vi "DAQNavi Read (Counter 1D Count Value NChan 1Samp).vi"(8 "error in (no error)":errorcluster, 11 "task in":i32) -> (0 "error out":errorcluster, 2 "data":i32[](array[numeric]), 3 "task out":i32)   [LabVIEW 2020]
uses:
  DAQNavi_LV.dll
panel:
  in  "timeout":dbl=10.0
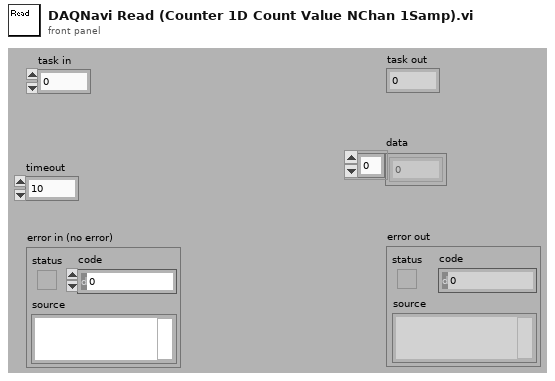
[diagram p1: front panel]
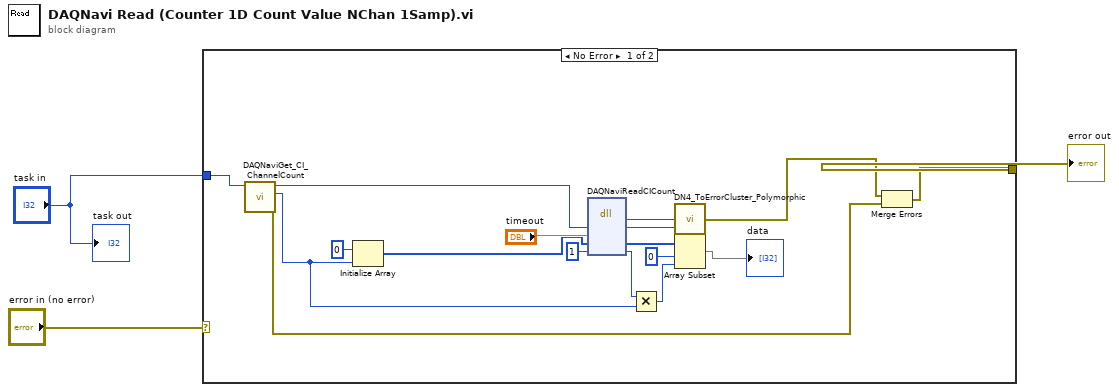
[diagram p0: block diagram]
diagram:
  n1 = case shown="No Error" "error in (no error)" {
    selector: "error in (no error)" -> [_ w21]
    tunnel: "task in" -> [w20 _]
    tunnel: [w4 w21] -> w1
    frame No Error {
      n2 = call "DAQNaviGet_CI_ChannelCount.vi"("task in"=w20) -> ("error out"=w5:errorcluster, "channel count"=w8:i32, "task out"=w13:i32)  [unwired: 1 in, 7 out]
      n3 = Initialize Array(0 ("element"), w8) -> (w11:i32[])
      n4 = dll-call lib="DAQNavi_LV.dll" fn="DAQNaviReadCICount"("taskID"=w13, "timeout"="timeout", "count"=w11, "samples"=u32 1) -> ("return type"=w19:i32, "taskID"=w14:i32, "count"=w17:i32[], "samples"=w9:u32)  [unwired: 4 in, 2 out]
      n5 = Multiply(x=w9, y=w8) -> (x*y=w10:u32)
      n6 = call "DN4_ToErrorCluster_Polymorphic.vi"("task id"=w14, "error code"=w19) -> ("error out"=w6:errorcluster)  [unwired: 3 out]
      n7 = Array Subset(array=w17, index=0, length=w10) -> (→"data":i32[])
      n8 = Merge Errors(w6, w5) -> (w4:errorcluster)
    }
    frame Error {
    }
  }
  "error out" <- w1
  "task out" <- "task in"
